vi "Dip Stamp Precheck.vi"(8 "error in (no error)":errorcluster, 11 "GrabberTool Class in":refnum<class "GrabberTool Class.lvclass">) -> (0 "error out":errorcluster, 3 "GrabberTool Class out":refnum<class "GrabberTool Class.lvclass">)   [LabVIEW 2011, in "GrabberTool Class.lvclass"]
uses:
  GrabberTool Class.lvclass
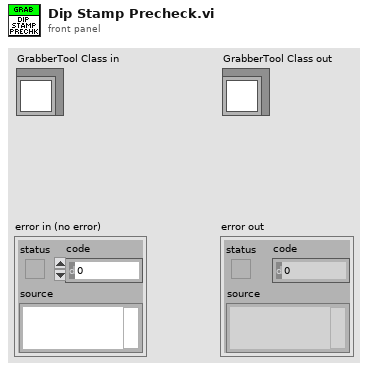
[diagram p1: front panel]
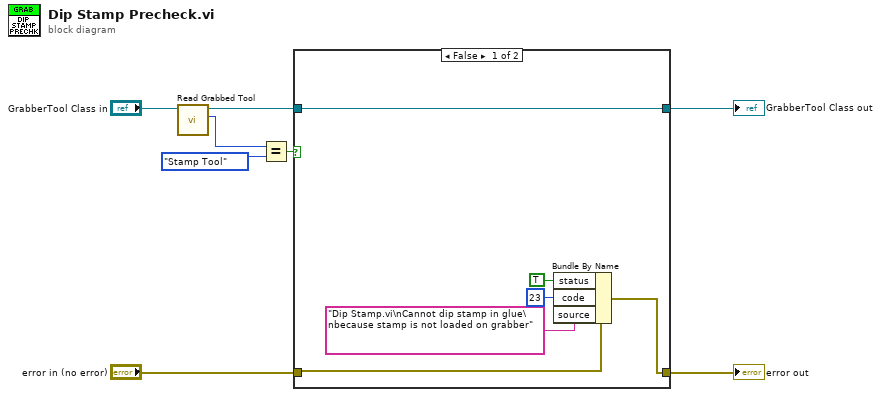
[diagram p0: block diagram]
diagram:
  n1 = call "Read Grabbed Tool.vi"("GrabberTool Class in"="GrabberTool Class in") -> ("Grabbed Tool"=w5:enum16{"Weight Tool", "Stamp Tool", "Nothing"}, "GrabberTool Class out"=w6:refnum<class "GrabberTool Class.lvclass">)  [unwired: 8 in, 1 out]
  n2 = Equal?(x=w5, y=enum16{"Weight Tool", "Stamp Tool", "Nothing"}."Stamp Tool") -> (x = y?=w3:bool)
  n3 = case shown="False" w3 {
    tunnel: [w13 w15] -> w8
    tunnel: [w14 w16] -> w1
    tunnel: w6 -> [w14 w16]
    tunnel: "error in (no error)" -> [w12 w15]
    frame False {
      n4 = Bundle By Name(cluster=w12, "status"=TRUE, "code"=23, "source"="Dip Stamp.vi\nCannot dip stamp in glue\nbecause stamp is not loaded on grabber") -> (w13:errorcluster)
    }
    frame True {
    }
  }
  "error out" <- w8
  "GrabberTool Class out" <- w1
